vi "WriteMWStageSettings.vi"(1 "error in (no error)":errorcluster) -> (0 "error out":errorcluster)   [LabVIEW 2009]
uses:
  MW settings.ctl
  <vilib>/Utility/config.llb/NI_LVConfig.lvlib
panel:
  out "MW Settings":T1={"Controller ID"=1, "Interface"={"Interface"=10, "COM-Port"=10, "Baudrate"=0, "I/O-Adress (ISA)"=0}, "Stage"={"Pitch [mm/U]"={"X"=10.0, "Y"=10.0, "Z"=0.0, "A"=0.0}, "Joy Velocity [U/s]"={"X"=10.0, "Y"=10.0, "Z"=0.0, "A"=0.0}, "Acceleration [m/s²]"={"X"=10.0, "Y"=10.0, "Z"=0.0, "A"=0.0}}} {"Stage"."Acceleration [m/s²]"."A" format="%.2f"; "Stage"."Acceleration [m/s²]"."Z" format="%.2f"; "Stage"."Acceleration [m/s²]"."Y" format="%.2f"; "Stage"."Acceleration [m/s²]"."X" min=0.0 max=10.0 format="%.2f"; "Stage"."Pitch [mm/U]"."A" format="%.2f"; "Stage"."Pitch [mm/U]"."Z" format="%.2f"; "Stage"."Pitch [mm/U]"."Y" format="%.2f"; "Stage"."Pitch [mm/U]"."X" format="%.2f"; "Stage"."Joy Velocity [U/s]"."A" format="%.2f"; "Stage"."Joy Velocity [U/s]"."Z" format="%.2f"; "Stage"."Joy Velocity [U/s]"."Y" format="%.2f"; "Stage"."Joy Velocity [U/s]"."X" format="%.2f"; "Interface"."Interface" items=["", "RS232", "", "ISA", "PCI"]}
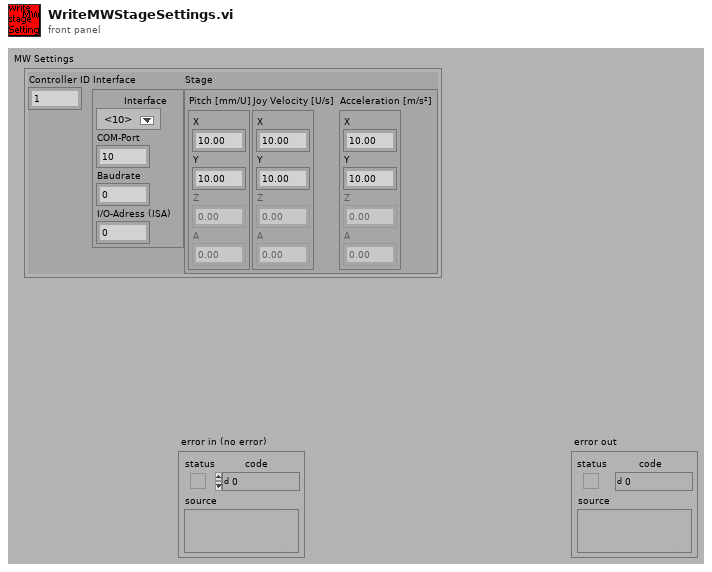
[diagram p1: front panel]
types:
  T1 = typedef "MW settings.ctl" = cluster{"Controller ID":i32, "Interface":cluster{"Interface":u32, "COM-Port":u32, "Baudrate":u32, "I/O-Adress (ISA)":u32}, "Stage":cluster{"Pitch [mm/U]":cluster{"X":dbl, "Y":dbl, "Z":dbl, "A":dbl}, "Joy Velocity [U/s]":cluster{"X":dbl, "Y":dbl, "Z":dbl, "A":dbl}, "Acceleration [m/s²]":cluster{"X":dbl, "Y":dbl, "Z":dbl, "A":dbl}}}
  T2 = typedef "NI_LVConfig.lvlib/Config Data RefNum.ctl" = refnum<k1>
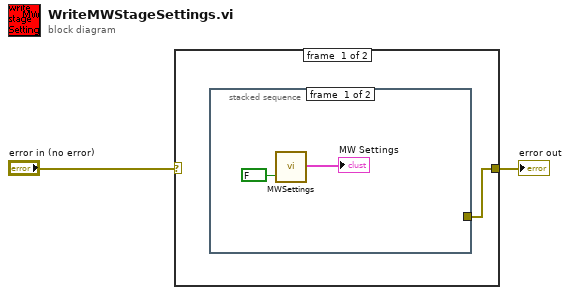
[diagram p0: block diagram]
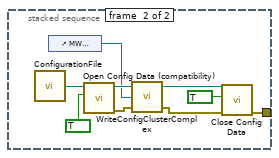
[diagram p2: hidden frame]
diagram:
  n1 = case shown="No Error" "error in (no error)" {
    selector: "error in (no error)" -> [_ w15]
    tunnel: [w3 w15] -> w1
    frame #0 {
      n2 = stacked-sequence {
        tunnel: [_ w6] -> w3
        frame #0 {
          n3 = call "MWSettings.vi"("set?"=FALSE) -> ("MW Settings out"=→"MW Settings":T1)  [unwired: 1 in]
        }
        frame #1 {
          n4 = call "ConfigurationFile.vi"() -> ("Configuration File (output)"=w14:path)  [unwired: 2 in]
          n5 = control-ref of="MW Settings"() -> (w7:refnum<vi>)
          n6 = call <vilib>:"Open Config Data (compatibility).vi"("create file if necessary (T)"=TRUE ("create file if necessary? (T)"), "configuration file path"=w14) -> ("error out"=w11:errorcluster, "refnum"=w12:T2)  [unwired: 7 in, 1 out]
          n7 = call "WriteConfigClusterComplex.vi"("error in (no error)"=w11, "Cluster 2"=w7, "Configfile input"=w12) -> ("error out"=w8:errorcluster, "refnum out"=w9:T2)  [unwired: 1 in]
          n8 = call "Close Config Data.vi"("error in (no error)"=w8, "write configuration file? (T)"=TRUE ("write configuration file? (F)"), "refnum"=w9) -> ("error out"=w6:errorcluster)  [unwired: 8 in]
        }
      }
    }
    frame #1 {
    }
  }
  "error out" <- w1
